vi "Show Panel.vi"(8 "error in (no error)":errorcluster, 10 "Panel In":refnum<class "Panel.lvclass">, 11 "Manager in":refnum<class "Manager.lvclass">) -> (0 "error out":errorcluster, 2 "Panel":refnum<class "Panel.lvclass">, 3 "Manager out":refnum<class "Manager.lvclass">)   [LabVIEW 2020, in "OOPanel.lvlib" / "Manager.lvclass"]
uses:
  Manager.lvclass
  Panel/Panel.lvclass
  Visibility State.ctl
  OOPanel.lvlib
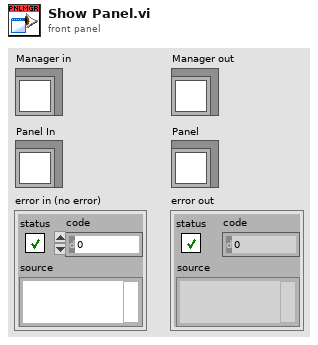
[diagram p1: front panel]
types:
  T1 = typedef "OOPanel.lvlib/Visibility State.ctl" = enum16{"Idle", "Closed", "Hidden", "Visible", "Subpanel", "Hidden Subpanel"}
  T2 = enum32{"Invalid", "Standard", "Closed", "Hidden", "Minimized", "Maximized"}
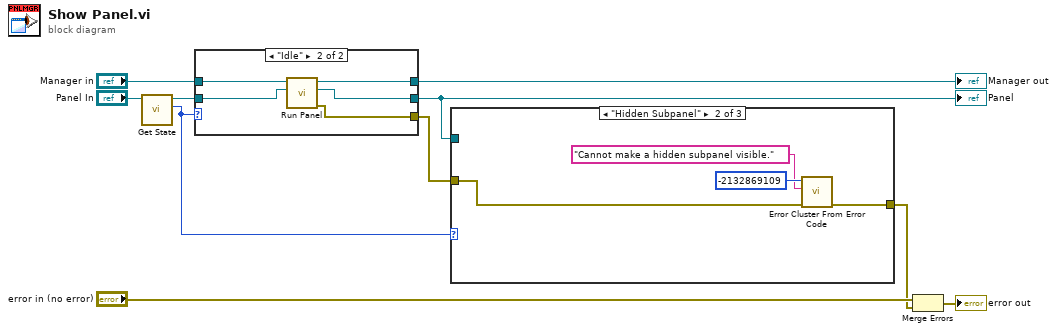
[diagram p0: block diagram]
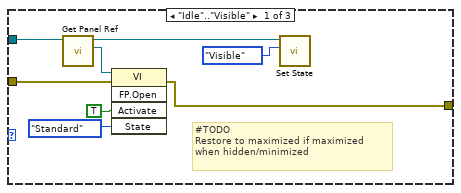
[diagram p3: hidden frame]
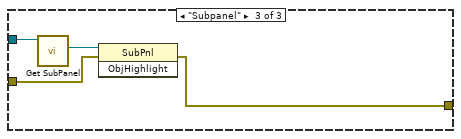
[diagram p4: hidden frame]
diagram:
  n1 = call "Get State.vi"("Panel in"="Panel In") -> ("State"=w5:T1, "Panel out"=w6:refnum<class "Panel.lvclass">)  [unwired: 8 in, 1 out]
  n2 = case shown="\"Idle\"" w5 {
    tunnel: w6 -> [w12 w16]
    tunnel: "Manager in" -> [w11 w17]
    tunnel: [w12 w15] -> w1
    tunnel: [w11 w14] -> w3
    tunnel: [_ w13] -> w2
    frame "Closed".."Hidden Subpanel" {
    }
    frame "Idle" {
      n3 = call "Run Panel.vi"("Panel In"=w16, "Manager in"=w17) -> ("error out"=w13:errorcluster, "Panel"=w15:refnum<class "Panel.lvclass">, "Manager out"=w14:refnum<class "Manager.lvclass">)  [unwired: 7 in]
    }
  }
  "Manager out" <- w3
  "Panel" <- w1
  n4 = case shown="\"Hidden Subpanel\"" w5 {
    tunnel: w1 -> [w25 _ w33]
    tunnel: [w21 w29 w31] -> w8
    tunnel: w2 -> [w20 w26 w30]
    frame "Idle".."Visible" {
      # "#TODO\nRestore to maximized if maximized when hidden/minimized"
      n5 = call "Get Panel Ref.vi"("Panel in"=w25) -> ("Panel Ref"=w24:refnum<vi>, "Panel out"=w19:refnum<class "Panel.lvclass">)  [unwired: 8 in, 1 out]
      n6 = invoke class="VI" method="FP.Open"(reference=w24, error in=w20, "Activate"=TRUE ("Activate?"), "State"=T2."Standard" ("Front Panel Window:State")) -> (error out=w21:errorcluster)  [unwired: 1 in, 4 out]
      n7 = call "Set State.vi"("State"=Visibility_State."Visible", "Panel in"=w19) -> ()  [unwired: 8 in, 2 out]
    }
    frame "Hidden Subpanel" {
      n8 = call <vilib>:"Error Cluster From Error Code.vi"("error in (no error)"=w26, "error message (\"\")"="Cannot make a hidden subpanel visible." ("error message (\"\")"), "error code (0)"=-2132869109) -> ("error out"=w29:errorcluster)  [unwired: 6 in]
    }
    frame "Subpanel" {
      n9 = call "Get SubPanel.vi"("Panel in"=w33) -> ("SubPanel"=w32:refnum<vi>)  [unwired: 8 in, 2 out]
      n10 = invoke class="SubPnl" method="ObjHighlight"(reference=w32, error in=w30) -> (error out=w31:errorcluster)  [unwired: 1 in, 2 out]
    }
  }
  n11 = Merge Errors("error in (no error)", w8) -> (→"error out":errorcluster)
